vi "Periodic Tasks.vi"(8 "error in":errorcluster) -> ()   [LabVIEW 2015]
doc: "This VI runs in parallel to other tasks. It can contain as many user-defined periodic loops as you need. These can carry out PID or other sorts of timed response."
uses:
  <vilib>/Rock Robotics/WPI/DriverStation/WPI_DriverStationRobotMode2.ctl
  <vilib>/Rock Robotics/WPI/Solenoid/WPI_SolenoidValue.ctl
  <vilib>/Rock Robotics/WPI/Utilities/WPI_GetSetVariantRefNum.vi
  Robot Global Data.vi
  <vilib>/Rock Robotics/WPI/Solenoid/WPI_SolenoidSetEnum.vi
  <vilib>/Rock Robotics/Network Tables/NT Write Boolean.vi
  <vilib>/Rock Robotics/Network Tables/NT Write Number.vi
  <vilib>/Rock Robotics/Network Tables/NT Read Boolean.vi
  NavX/navX Library v2/navX Library v2.lvlib
panel:
  out "12 (Shooter angle)":dbl
  out "Shooter 2":dbl
  out "Shooter 1":dbl
  out "Energy (J)":dbl
  out "Power (W)":dbl
  out "15":dbl
  out "0":dbl
  out "14":dbl
  out "1":dbl
  out "current (A)":dbl
  out "Loop Time":u32
  in  "Roll":dbl=3.0
  in  "Pitch":dbl=3.0
  out "Value":bool
  out "Enum":T1(ring)
  out "isFlat":bool
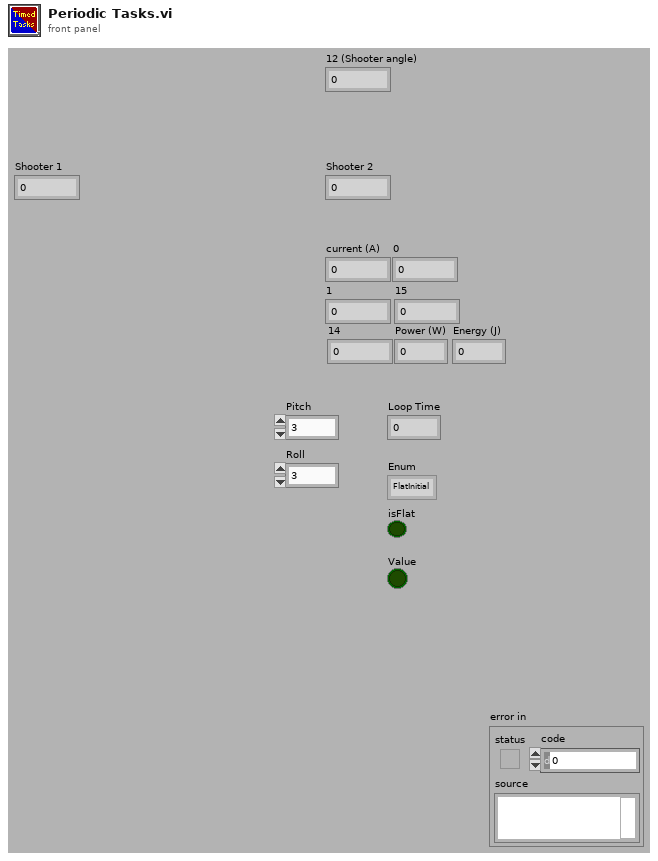
[diagram p1: front panel]
types:
  T1 = enum16{"FlatInitial", "AngleUp", "AngleDown", "FlatFinal"}
  T2 = typedef "WPI_RobotDriveDevRef.ctl" = cluster{"DevStatus":errorcluster, "Motors[]":T3[], "Square Inputs":bool, "Max Output":dbl}
  T3 = typedef "WPI_MotorControlDeviceRef.ctl" = cluster{"DeviceStatus":errorcluster, "Type":T4, "PWM":cluster{"PWM Channel":T5, "DeadBand":T6}, "CAN":cluster{"Device Number":u8, "Control Mode":T7, "Semaphore":T8, "Max Vout":dbl, "TalonSRX Control Mode":T9}, "Invert":bool}
  T4 = typedef "WPI_MotorControlType.ctl" = enum16{"PWM", "CAN", "CANTalonSRX"}
  T5 = typedef "FPGA_DIOPWMChannel.ctl" = enum8{"PWM 0", "PWM 1", "PWM 2", "PWM 3", "PWM 4", "PWM 5", "PWM 6", "PWM 7", "PWM 8", "PWM 9", "PWM MXP 0", "PWM MXP 1", "PWM MXP 2", "PWM MXP 3", "PWM MXP 4", "PWM MXP 5", "PWM MXP 6", "PWM MXP 7", "PWM MXP 8", "PWM MXP 9", "Invalid"}
  T6 = typedef "WPI_PWMDeadband.ctl" = cluster{"Name":string, "maxPositivePwm":i32, "minPositivePwm":i32, "centerPwm":i32, "maxNegativePwm":i32, "minNegativePwm":i32, "angularRange":u16}
  T7 = typedef "WPI_CANJaguar_ControlMode.ctl" = enum8{"Percent VBus", "Current", "Speed", "Position", "Voltage"}
  T8 = typedef "Semaphore RefNum" = refnum<k1>
  T9 = typedef "WPI_CANTalonSRX_APIControlMode.ctl" = enum8{"Percent VBus", "Speed", "Position", "Slave", "Unchanged / Invalid", "Voltage Compensation", "Current", "Motion Profile"}
  T10 = typedef "WPI_DigitalInputDevRef.ctl" = cluster{"DevStatus":errorcluster, "DIO Channel":T11}
  T11 = typedef "FPGA_DIOChannel.ctl" = enum8{"DIO 0", "DIO 1", "DIO 2", "DIO 3", "DIO 4", "DIO 5", "DIO 6", "DIO 7", "DIO 8", "DIO 9", "DIO MXP 0", "DIO MXP 1", "DIO MXP 2", "DIO MXP 3", "DIO MXP 4", "DIO MXP 5", "DIO MXP 6", "DIO MXP 7", "DIO MXP 8", "DIO MXP 9", "DIO MXP 10", "DIO MXP 11", "DIO MXP 12", "DIO MXP 13", "DIO MXP 14", "DIO MXP 15", "Invalid"}
  T12 = typedef "WPI_SolenoidDevRef.ctl" = cluster{"DevStatus":errorcluster, "Pneumatics Control Module":u8, "Forward Solenoid Channel":T13, "Reverse Solenoid Channel":T13}
  T13 = typedef "WPI_SolenoidChannel.ctl" = enum8{"Solenoid 0", "Solenoid 1", "Solenoid 2", "Solenoid 3", "Solenoid 4", "Solenoid 5", "Solenoid 6", "Solenoid 7", "Invalid"}
  T14 = typedef "WPI_EncoderDevRef.ctl" = cluster{"DevStatus":errorcluster, "EncoderIndex":T15, "CounterIndex":T16, "DistancePerCount":dbl, "Decoding Type":T17}
  T15 = typedef "FPGA_EncoderIdx.ctl" = enum8{"Enc 0", "Enc 1", "Enc 2", "Enc 3", "Enc 4", "Enc 5", "Enc 6", "Enc 7", "Invalid"}
  T16 = typedef "FPGA_CounterCtrSystemIndex.ctl" = enum8{"Ctr 0", "Ctr 1", "Ctr 2", "Ctr 3", "Ctr 4", "Ctr 5", "Ctr 6", "Ctr 7", "Invalid"}
  T17 = typedef "WPI_EncoderType.ctl" = enum16{"1x", "2x", "4x"}
  T18 = typedef "navX Library v2.lvlib/Z900_navX_DeviceTypeDef.ctl" = cluster{"Interface":cluster{"Protocol":T19, "Update Rate (4Hz-60Hz)":u8, "navX Open TypeDef":variant}, "Notify Packet":refnum<notifier>, "Loop VI Refnum":refnum<vi>, "Ready to Close Occurrence Refnum":refnum<k4>}
  T19 = typedef "navX Library v2.lvlib/Z900_navX_ProtocolTypeDef.ctl" = enum16{"SERIAL", "I2C", "SPI"}
  T20 = typedef "WPI_SolenoidValue.ctl" = enum16{"Off", "On", "Forward", "Reverse"}
  T21 = typedef "WPI_DriverStationRobotMode2.ctl" = enum16{"Autonomous Disabled", "Autonomous Enabled", "Teleop Disabled", "Teleop Enabled", "Disconnected", "Finish", "Test Disabled", "Test Enabled", "Emergency Stopped"}
  T22 = typedef "WPI_GyroDevRef.ctl" = cluster{"DevStatus":errorcluster, "Analog Channel":T23, "Offset":dbl, "Gain (VoltsPerDegree/Second)":dbl, "Gyro Type":enum16{"Analog", "XRS450"}, "Handle":i32, "SPI Bus":T24, "Device Found":bool, "Sample Rate":dbl, "Calibrate On Open":bool}
  T23 = typedef "FPGA_AIChannel.ctl" = enum8{"AI 0", "AI 1", "AI 2", "AI 3", "AI MXP 0", "AI MXP 1", "AI MXP 2", "AI MXP 3", "Invalid"}
  T24 = typedef "spi_bus.ctl" = enum16{"SPI On-Board, CS0", "SPI On-Board, CS1", "SPI On-Board, CS2", "SPI On-Board, CS3", "SPI MXP", "Invalid"}
  T25 = cluster{"Velocity X":dbl, "Velocity Y":dbl, "Velocity Z":dbl, "Displacement X":dbl, "Displacement Y":dbl, "Displacement Z":dbl}
  T26 = cluster{"Yaw":dbl, "Roll":dbl, "Pitch":dbl, "Heading":dbl, "Fused Heading":dbl}
  T27 = enum16{"Empty", "Suck", "Hold", "LowGoal", "HighGoal", "BumperShot", "Shoot", "Dwell"}
  T28 = enum16{"ResetBack", "EmergencyManualControl", "ResetForward", "Hold", "Reset", "ManualControl"}
  T29 = cluster{"LinearAcceleration X":dbl, "LinearAcceleration Y":dbl, "LinearAcceleration Z":dbl}
  T30 = enum16{"ResetBack", "ResetForward", "Reset", "Hold", "HighGoal", "LowGoal", "BumperShot", "EmergencyManualControl"}
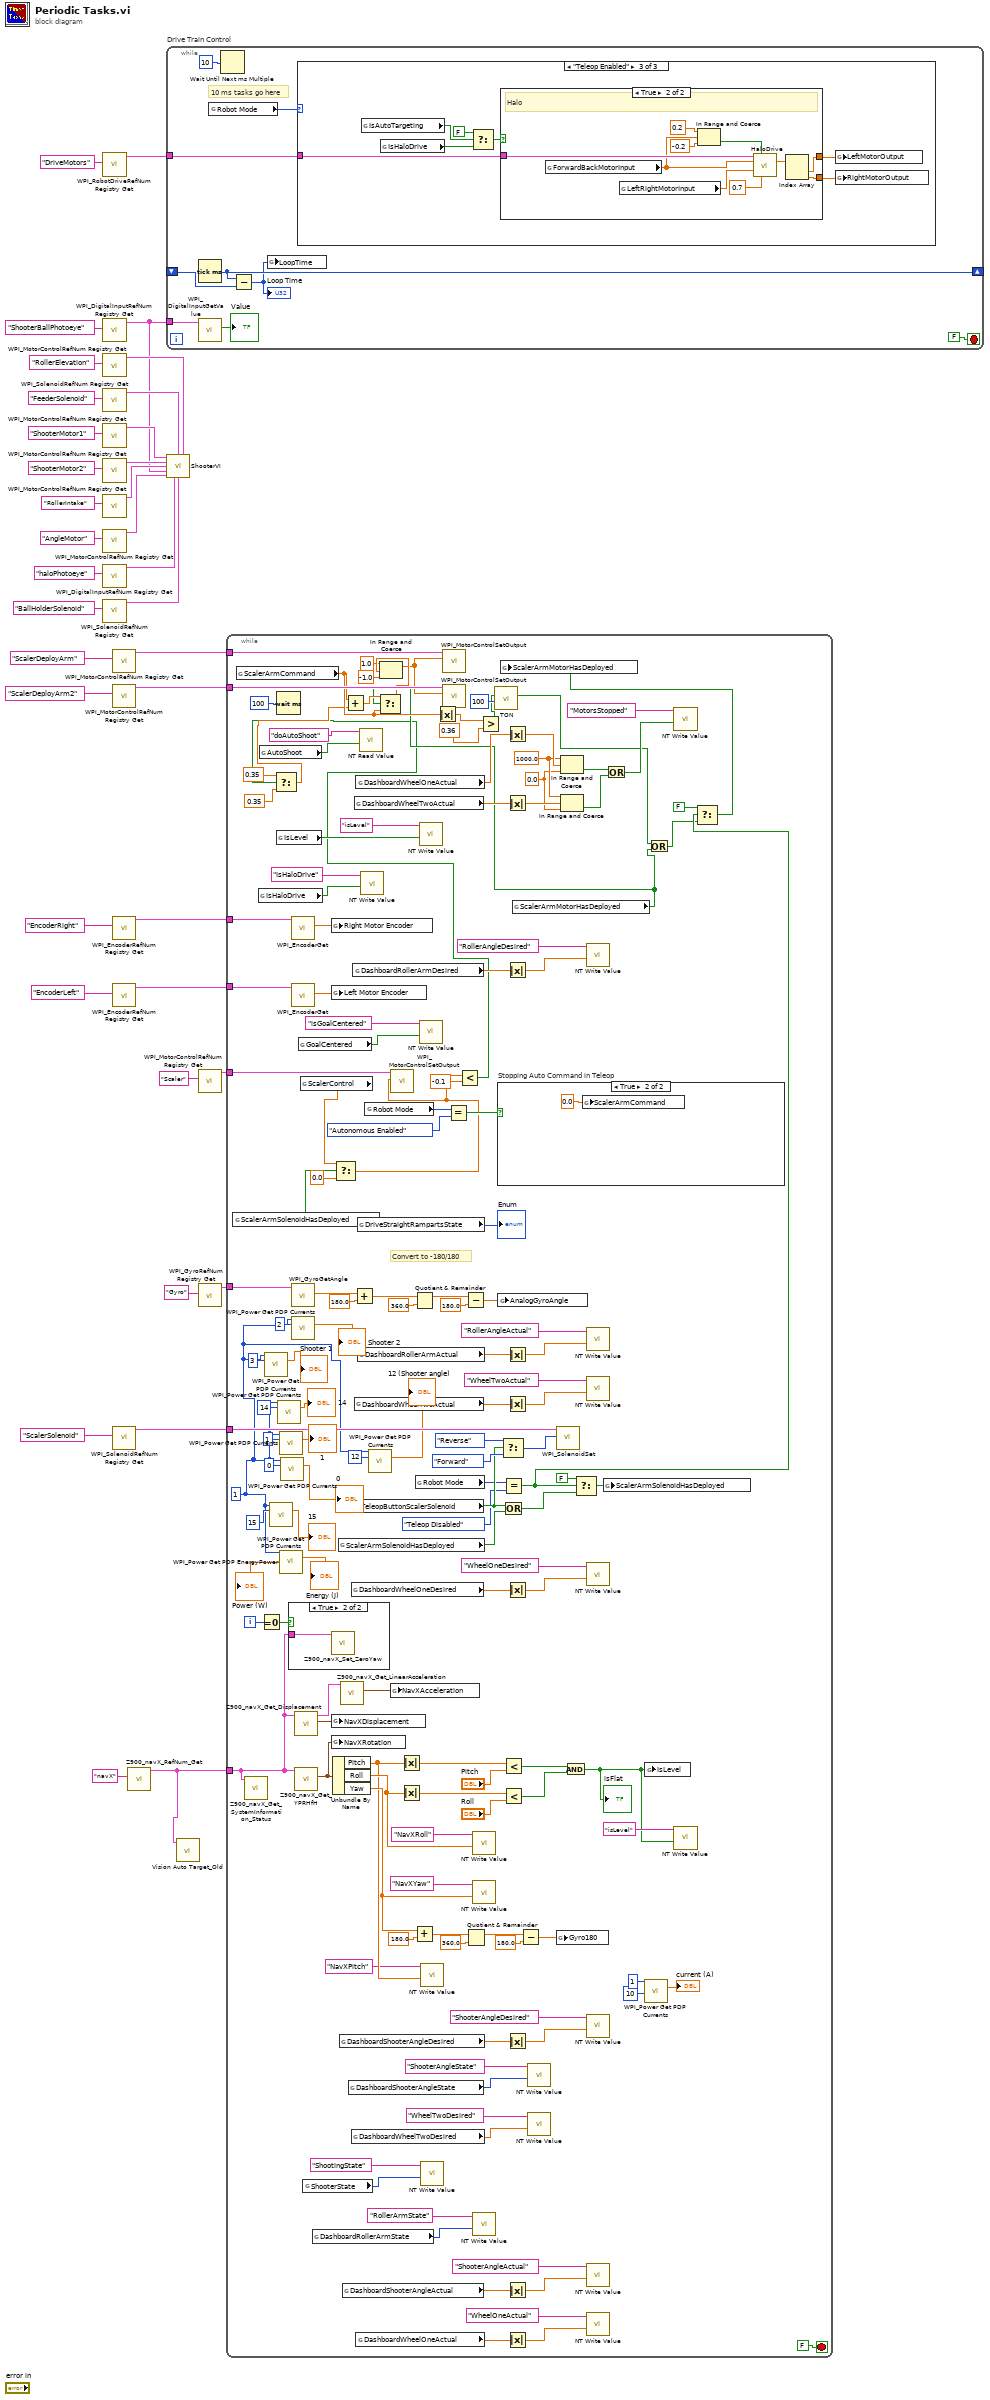
[diagram p0: block diagram]
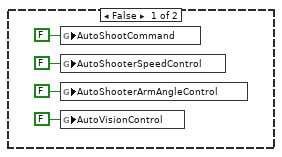
[diagram p2: hidden frame]
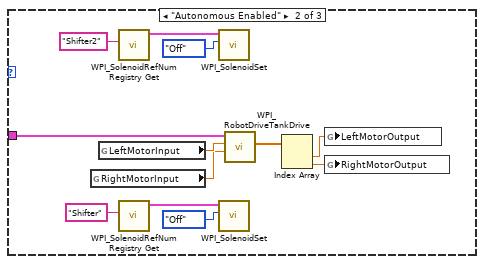
[diagram p5: hidden frame]
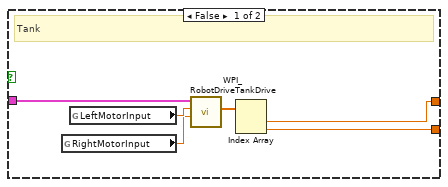
[diagram p6: hidden frame]
diagram:
  n1 = call <vilib>:"WPI_RobotDriveRefNum Registry Get.vi"("refnum name"="DriveMotors") -> ("RobotDriveDevRef"=w35:T2)  [unwired: 9 in, 1 out]
  n2 = call <vilib>:"WPI_DigitalInputRefNum Registry Get.vi"("refnum name"="ShooterBallPhotoeye") -> ("DigitalInputDevRef"=w1:T10)  [unwired: 9 in, 1 out]
  n3 = call <vilib>:"WPI_MotorControlRefNum Registry Get.vi"("refnum name"="RollerElevation") -> ("MotorControlDevRef"=w23:T3)  [unwired: 9 in, 1 out]
  n4 = call <vilib>:"WPI_SolenoidRefNum Registry Get.vi"("refnum name"="FeederSolenoid") -> ("SolenoidDevRef"=w19:T12)  [unwired: 9 in, 1 out]
  n5 = call <vilib>:"WPI_MotorControlRefNum Registry Get.vi"("refnum name"="ShooterMotor1") -> ("MotorControlDevRef"=w22:T3)  [unwired: 9 in, 1 out]
  n6 = call <vilib>:"WPI_MotorControlRefNum Registry Get.vi"("refnum name"="ShooterMotor2") -> ("MotorControlDevRef"=w21:T3)  [unwired: 9 in, 1 out]
  n7 = call <vilib>:"WPI_MotorControlRefNum Registry Get.vi"("refnum name"="RollerIntake") -> ("MotorControlDevRef"=w20:T3)  [unwired: 9 in, 1 out]
  n8 = call <vilib>:"WPI_MotorControlRefNum Registry Get.vi"("refnum name"="AngleMotor") -> ("MotorControlDevRef"=w17:T3)  [unwired: 9 in, 1 out]
  n9 = call <vilib>:"WPI_DigitalInputRefNum Registry Get.vi"("refnum name"="haloPhotoeye") -> ("DigitalInputDevRef"=w3:T10)  [unwired: 9 in, 1 out]
  n10 = call <vilib>:"WPI_SolenoidRefNum Registry Get.vi"("refnum name"="BallHolderSolenoid") -> ("SolenoidDevRef"=w10:T12)  [unwired: 9 in, 1 out]
  n11 = call <vilib>:"WPI_MotorControlRefNum Registry Get.vi"("refnum name"="ScalerDeployArm") -> ("MotorControlDevRef"=w16:T3)  [unwired: 9 in, 1 out]
  n12 = call <vilib>:"WPI_MotorControlRefNum Registry Get.vi"("refnum name"="ScalerDeployArm2") -> ("MotorControlDevRef"=w5:T3)  [unwired: 9 in, 1 out]
  n13 = call <vilib>:"WPI_EncoderRefNum Registry Get.vi"("refnum name"="EncoderRight") -> ("EncoderDevRef"=w31:T14)  [unwired: 9 in, 1 out]
  n14 = call <vilib>:"WPI_EncoderRefNum Registry Get.vi"("refnum name"="EncoderLeft") -> ("EncoderDevRef"=w32:T14)  [unwired: 9 in, 1 out]
  n15 = call <vilib>:"WPI_SolenoidRefNum Registry Get.vi"("refnum name"="ScalerSolenoid") -> ("SolenoidDevRef"=w7:T12)  [unwired: 9 in, 1 out]
  n16 = call "Z900_navX_RefNum_Get.vi"("refnum name"="navX") -> ("navX Device"=w2:T18)  [unwired: 9 in, 1 out]
  n17 = while "Drive Train Control" {
    tunnel: w35 -> [w44]
    tunnel: w1 -> [w42]
    shift-right: [w39] -> _
    shift-left: _ -> [w40]
    stop <- FALSE stop-if-true
    # "10 ms tasks go here"
    n18 = Tick Count (ms)() -> (millisecond timer value=w39:u32)
    n19 = call <vilib>:"WPI_DigitalInputGetValue.vi"("DigitalInputDevRef"=w42) -> ("Value"=→"Value":bool)  [unwired: 8 in, 2 out]
    n20 = global read "Robot Global Data.vi" "Robot Mode"() -> (w43:T21)
    n21 = Wait Until Next ms Multiple(millisecond multiple=u32 10 ("milliseconds to wait")) -> ()  [unwired: 1 out]
    n22 = Subtract(x=w39, y=w40) -> (x-y=w38:u32)
    "Loop Time" <- w38
    n23 = global write "Robot Global Data.vi" "LoopTime"(w38) -> ()
    n24 = case shown="\"Teleop Enabled\"" w43 {
      tunnel: w44 -> [_ w57 w64]
      frame "Autonomous Disabled", "Teleop Disabled", Default {
      }
      frame "Autonomous Enabled" {
        n25 = global read "Robot Global Data.vi" "RightMotorInput"() -> (w49:dbl)
        n26 = global read "Robot Global Data.vi" "LeftMotorInput"() -> (w50:dbl)
        n27 = call <vilib>:"WPI_SolenoidRefNum Registry Get.vi"("refnum name"="Shifter2") -> ("SolenoidDevRef"=w52:T12)  [unwired: 9 in, 1 out]
        n28 = call <vilib>:"WPI_SolenoidRefNum Registry Get.vi"("refnum name"="Shifter") -> ("SolenoidDevRef"=w51:T12)  [unwired: 9 in, 1 out]
        n29 = call-poly <vilib>:"WPI_SolenoidSet.vi"("Value"=WPI_SolenoidValue."Off", "SolenoidDevRef"=w52) -> ()  [unwired: 8 in, 2 out]
        n30 = call-poly <vilib>:"WPI_SolenoidSet.vi"("Value"=WPI_SolenoidValue."Off", "SolenoidDevRef"=w51) -> ()  [unwired: 8 in, 2 out]
        n31 = call <vilib>:"WPI_RobotDriveTankDrive.vi"("Right axis value"=w49, "Left axis value"=w50, "RobotDriveDevRef"=w57) -> ("Motor Values"=w48:dbl[])  [unwired: 6 in, 2 out]
        n32 = Index Array(array=w48) -> (element #1=w47:dbl, element #2=w46:dbl)  [unwired: 2 in]
        n33 = global write "Robot Global Data.vi" "LeftMotorOutput"(w47) -> ()
        n34 = global write "Robot Global Data.vi" "RightMotorOutput"(w46) -> ()
      }
      frame "Teleop Enabled" {
        n35 = global read "Robot Global Data.vi" "IsAutoTargeting"() -> (w61:bool)
        n36 = global read "Robot Global Data.vi" "IsHaloDrive"() -> (w59:bool)
        n37 = Select(t=FALSE, s=w61, f=w59) -> (s? t:f=w58:bool)
        n38 = case shown="True" w58 {
          tunnel: w64 -> [w68 w80]
          tunnel: [w67 w72] -> w63
          tunnel: [w66 w71] -> w62
          frame False {
            # "Tank"
            n39 = global read "Robot Global Data.vi" "RightMotorInput"() -> (w69:dbl)
            n40 = global read "Robot Global Data.vi" "LeftMotorInput"() -> (w70:dbl)
            n41 = call <vilib>:"WPI_RobotDriveTankDrive.vi"("Right axis value"=w69, "Left axis value"=w70, "RobotDriveDevRef"=w68) -> ("Motor Values"=w65:dbl[])  [unwired: 6 in, 2 out]
            n42 = Index Array(array=w65) -> (element #1=w67:dbl, element #2=w66:dbl)  [unwired: 2 in]
          }
          frame True {
            # "Halo"
            n43 = global read "Robot Global Data.vi" "ForwardBackMotorInput"() -> (w74:dbl)
            n44 = global read "Robot Global Data.vi" "LeftRightMotorInput"() -> (w75:dbl)
            n45 = In Range and Coerce(upper limit=0.2, x=w74, lower limit=-0.2) -> (In Range?=w76:bool)  [unwired: 1 out]
            n46 = call "HaloDrive.vi"("RobotDriveDevRef 2"=w80, "QwikTurnButton"=w76, "Left axis value"=w74, "Right axis value"=w75, "Sensitivity"=0.7) -> ("Motor Values"=w73:dbl[])  [unwired: 6 in, 4 out]
            n47 = Index Array(array=w73) -> (element #1=w72:dbl, element #2=w71:dbl)  [unwired: 2 in]
          }
        }
        n48 = global write "Robot Global Data.vi" "LeftMotorOutput"(w63) -> ()
        n49 = global write "Robot Global Data.vi" "RightMotorOutput"(w62) -> ()
      }
    }
  }
  n50 = call "ShooterVI.vi"("Shooter Motor 1"=w22, "ShooterSolenoid"=w19, "Roller Angle Motor"=w23, "Shooter Motor 2"=w21, "Roller Intake Motor"=w20, "Ball Detector Photoeye"=w1, "ShooterAngleMotor"=w17, "Halo Photoeye"=w3, "BallHolderSolenoid"=w10) -> ()  [unwired: 7 in]
  n51 = call "Vision Auto Target_Old.vi"("navX Device"=w2) -> ()  [unwired: 11 in]
  n52 = call <vilib>:"WPI_MotorControlRefNum Registry Get.vi"("refnum name"="Scaler") -> ("MotorControlDevRef"=w14:T3)  [unwired: 9 in, 1 out]
  n53 = call <vilib>:"WPI_GyroRefNum Registry Get.vi"("refnum name"="Gyro") -> ("GyroDevRef"=w13:T22)  [unwired: 9 in, 1 out]
  n54 = while {
    tunnel: w32 -> [w228]
    tunnel: w31 -> [w229]
    tunnel: w2 -> [w150]
    tunnel: w16 -> [w173]
    tunnel: w14 -> [w172]
    tunnel: w13 -> [w158]
    tunnel: w7 -> [w146]
    tunnel: w5 -> [w145]
    i -> [w225]
    stop <- FALSE stop-if-true
    w83 = u8 1 ("Power Distribution Panel (0)")
    w139 = 0.0 ("lower limit")
    w140 = 1000.0
    # "Convert to -180/180"
    n55 = global read "Robot Global Data.vi" "ScalerArmSolenoidHasDeployed"() -> (w125:bool)
    n56 = global read "Robot Global Data.vi" "ScalerArmCommand"() -> (w112:dbl)
    n57 = call "Z900_navX_Get_SystemInformation_Status.vi"("navX Device"=w150) -> ()  [unwired: 7 in, 4 out]
    n58 = global read "Robot Global Data.vi" "IsHaloDrive"() -> (w226:bool)
    n59 = global read "Robot Global Data.vi" "AutoShoot"() -> (w185:bool)
    n60 = Equal To 0?(x=w225) -> (x = 0?=w224:bool)
    n61 = call <vilib>:"WPI_Power Get PDP Currents.vi"("Power Distribution Panel (0)"=w83, "PDP Channel"=3) -> ("current (A)"=→"Shooter 1":dbl)  [unwired: 11 in, 2 out]
    n62 = call <vilib>:"WPI_Power Get PDP Currents.vi"("Power Distribution Panel (0)"=w83, "PDP Channel"=15) -> ("current (A)"=→"15":dbl)  [unwired: 11 in, 2 out]
    n63 = global read "Robot Global Data.vi" "IsLevel"() -> (w183:bool)
    n64 = Wait (ms)(milliseconds to wait=u32 100) -> ()  [unwired: 1 out]
    n65 = call <vilib>:"WPI_Power Get PDP Currents.vi"("Power Distribution Panel (0)"=w83, "PDP Channel"=14) -> ("current (A)"=→"14":dbl)  [unwired: 11 in, 2 out]
    n66 = call <vilib>:"WPI_Power Get PDP Currents.vi"("Power Distribution Panel (0)"=w83, "PDP Channel"=1) -> ("current (A)"=→"1":dbl)  [unwired: 11 in, 2 out]
    n67 = call <vilib>:"WPI_Power Get PDP EnergyPower.vi"("Power Distribution Panel (0)"=w83) -> ("Energy (J)"=→"Energy (J)":dbl, "Power (W)"=→"Power (W)":dbl)  [unwired: 12 in, 1 out]
    n68 = call <vilib>:"WPI_Power Get PDP Currents.vi"("Power Distribution Panel (0)"=w83, "PDP Channel"=0) -> ("current (A)"=→"0":dbl)  [unwired: 11 in, 2 out]
    n69 = case shown="True" w224 {
      tunnel: w150 -> [_ w237]
      frame False {
      }
      frame True {
        n70 = call "Z900_navX_Set_ZeroYaw.vi"("navX Device"=w237) -> ()  [unwired: 9 in, 2 out]
      }
    }
    n71 = call <vilib>:"WPI_EncoderGet.vi"("EncoderDevRef"=w229) -> ("Distance"=w149:dbl)  [unwired: 5 in, 5 out]
    n72 = call <vilib>:"WPI_EncoderGet.vi"("EncoderDevRef"=w228) -> ("Distance"=w148:dbl)  [unwired: 5 in, 5 out]
    n73 = call <vilib>:"WPI_GyroGetAngle.vi"("GyroDevRef"=w158) -> ("Angle"=w152:dbl)  [unwired: 6 in, 4 out]
    n74 = call <vilib>:"WPI_Power Get PDP Currents.vi"("Power Distribution Panel (0)"=w83, "PDP Channel"=2) -> ("current (A)"=→"Shooter 2":dbl)  [unwired: 11 in, 2 out]
    n75 = call "Z900_navX_Get_Displacement.vi"("navX Device"=w150) -> ("Displacement"=w218:T25, "navX Device"=w216:T18)  [unwired: 7 in, 2 out]
    n76 = call "Z900_navX_Get_YPRHfH.vi"("navX Device"=w150) -> ("YRPHfH"=w223:T26)  [unwired: 7 in, 3 out]
    n77 = global read "Robot Global Data.vi" "GoalCentered"() -> (w187:bool)
    n78 = global read "Robot Global Data.vi" "ScalerControl"() -> (w123:dbl)
    n79 = global read "Robot Global Data.vi" "ShooterState"() -> (w204:T27)
    n80 = global read "Robot Global Data.vi" "DashboardRollerArmState"() -> (w203:T28)
    n81 = global write "Robot Global Data.vi" "Right Motor Encoder"(w149) -> ()
    n82 = global write "Robot Global Data.vi" "Left Motor Encoder"(w148) -> ()
    n83 = global write "Robot Global Data.vi" "NavXDisplacement"(w218) -> ()
    n84 = global write "Robot Global Data.vi" "NavXRotation"(w223) -> ()
    n85 = Unbundle By Name(w223) -> ("Pitch"=w175:dbl, "Roll"=w177:dbl, "Yaw"=w179:dbl)
    n86 = Select(t=w123, s=w125, f=0.0) -> (s? t:f=w106:dbl)
    n87 = global read "Robot Global Data.vi" "ScalerArmSolenoidHasDeployed"() -> (w131:bool)
    n88 = global read "Robot Global Data.vi" "DashboardShooterAngleDesired"() -> (w196:dbl)
    n89 = call "Z900_navX_Get_LinearAcceleration.vi"("navX Device"=w216) -> ("Linear Acceleration"=w217:T29)  [unwired: 7 in, 3 out]
    n90 = global read "Robot Global Data.vi" "DashboardShooterAngleActual"() -> (w195:dbl)
    n91 = global read "Robot Global Data.vi" "DashboardShooterAngleState"() -> (w202:T30)
    n92 = global read "Robot Global Data.vi" "DashboardWheelOneDesired"() -> (w201:dbl)
    n93 = global read "Robot Global Data.vi" "DashboardWheelTwoDesired"() -> (w199:dbl)
    n94 = global read "Robot Global Data.vi" "DashboardRollerArmDesired"() -> (w198:dbl)
    n95 = Add(x=w152, y=180.0) -> (x+y=w156:dbl)
    n96 = global read "Robot Global Data.vi" "TeleopButtonScalerSolenoid"() -> (w132:bool)
    n97 = global read "Robot Global Data.vi" "DashboardWheelTwoActual"() -> (w143:dbl)
    n98 = global read "Robot Global Data.vi" "DashboardWheelTwoActual"() -> (w194:dbl)
    n99 = global read "Robot Global Data.vi" "DashboardWheelOneActual"() -> (w144:dbl)
    n100 = global read "Robot Global Data.vi" "DashboardWheelOneActual"() -> (w200:dbl)
    n101 = global read "Robot Global Data.vi" "DriveStraightRampartsState"() -> (→"Enum":T1)
    n102 = global read "Robot Global Data.vi" "DashboardRollerArmActual"() -> (w197:dbl)
    n103 = call-poly <vilib>:"NT Read Value.vi"("Default Value"=w185, "Name"="doAutoShoot") -> ()  [unwired: 8 in, 2 out]
    n104 = call-poly <vilib>:"NT Write Value.vi"("Boolean"=w226, "Name"="IsHaloDrive") -> ()  [unwired: 9 in, 1 out]
    n105 = global read "Robot Global Data.vi" "Robot Mode"() -> (w169:T21)
    n106 = call <vilib>:"WPI_Power Get PDP Currents.vi"("Power Distribution Panel (0)"=w83, "PDP Channel"=12) -> ("current (A)"=→"12 (Shooter angle)":dbl)  [unwired: 11 in, 2 out]
    n107 = call <vilib>:"WPI_MotorControlSetOutput.vi"("Output"=w106, "MotorControlDevRef"=w172) -> ()  [unwired: 7 in, 3 out]
    n108 = global write "Robot Global Data.vi" "NavXAcceleration"(w217) -> ()
    n109 = Absolute Value(x=w175) -> (abs(x)=w222:dbl)
    n110 = Absolute Value(x=w177) -> (abs(x)=w220:dbl)
    n111 = Add(x=w179, y=180.0) -> (x+y=w192:dbl)
    n112 = Quotient & Remainder(x=w156, y=360.0) -> (x-y*floor(x/y)=w154:dbl)  [unwired: 1 out]
    n113 = global read "Robot Global Data.vi" "Robot Mode"() -> (w130:T21)
    n114 = call-poly <vilib>:"NT Write Value.vi"("Boolean"=w183, "Name"="isLevel") -> ()  [unwired: 9 in, 1 out]
    n115 = call-poly <vilib>:"NT Write Value.vi"("Boolean"=w187, "Name"="isGoalCentered") -> ()  [unwired: 9 in, 1 out]
    n116 = call-poly <vilib>:"NT Write Value.vi"("Numeric"=w175, "Name"="NavXPitch") -> ()  [unwired: 9 in, 1 out]
    n117 = call-poly <vilib>:"NT Write Value.vi"("Numeric"=w204, "Name"="ShootingState") -> ()  [unwired: 9 in, 1 out]
    n118 = Absolute Value(x=w112) -> (abs(x)=w114:dbl)
    n119 = Equal?(x=w169, y=WPI_DriverStationRobotMode2."Autonomous Enabled") -> (x = y?=w167:bool)
    n120 = Less?(x=w106, y=-0.1) -> (x < y?=w99:bool)
    n121 = Select(t=0.35, s=w99, f=0.35 ("y")) -> (s? t:f=w103:dbl)
    n122 = Add(x=w112, y=w103) -> (x+y=w113:dbl)
    n123 = Subtract(x=w154, y=180.0) -> (x-y=w151:dbl)
    n124 = Quotient & Remainder(x=w192, y=360.0) -> (x-y*floor(x/y)=w190:dbl)  [unwired: 1 out]
    n125 = call-poly <vilib>:"NT Write Value.vi"("Numeric"=w177, "Name"="NavXRoll") -> ()  [unwired: 9 in, 1 out]
    n126 = call-poly <vilib>:"NT Write Value.vi"("Numeric"=w179, "Name"="NavXYaw") -> ()  [unwired: 9 in, 1 out]
    n127 = call-poly <vilib>:"NT Write Value.vi"("Numeric"=w203, "Name"="RollerArmState") -> ()  [unwired: 9 in, 1 out]
    n128 = Greater?(x=w114, y=0.36 ("upper limit")) -> (0:w116:bool)
    n129 = call "TON.vi"("Delay (ms)"=u32 100, "Input"=w116) -> ("Output"=w121:bool)  [unwired: 9 in]
    n130 = case "Stopping Auto Command in Teleop" shown="True" w167 {
      frame False {
        n131 = global write "Robot Global Data.vi" "AutoShootCommand"(FALSE ("AutoShooterSpeedControl")) -> ()
        n132 = global write "Robot Global Data.vi" "AutoShooterSpeedControl"(FALSE ("AutoShooterSpeedControl")) -> ()
        n133 = global write "Robot Global Data.vi" "AutoShooterArmAngleControl"(FALSE ("AutoShooterSpeedControl")) -> ()
        n134 = global write "Robot Global Data.vi" "AutoVisionControl"(FALSE ("AutoVisionControl")) -> ()
      }
      frame True {
        n135 = global write "Robot Global Data.vi" "ScalerArmCommand"(0.0 ("ScalerArmCommand")) -> ()
      }
    }
    n136 = global write "Robot Global Data.vi" "AnalogGyroAngle"(w151) -> ()
    n137 = Select(t=WPI_SolenoidValue."Reverse" ("Value"), s=w132, f=WPI_SolenoidValue."Forward") -> (s? t:f=w133:T20)
    n138 = Equal?(x=w130, y=WPI_DriverStationRobotMode2."Teleop Disabled") -> (x = y?=w120:bool)
    n139 = Or(x=w132, y=w131) -> (x .or. y?=w128:bool)
    n140 = Less?(x=w222, y="Pitch") -> (x < y?=w221:bool)
    n141 = Less?(x=w220, y="Roll") -> (x < y?=w219:bool)
    n142 = Absolute Value(x=w144) -> (abs(x)=w142:dbl)
    n143 = Absolute Value(x=w143) -> (abs(x)=w141:dbl)
    n144 = Absolute Value(x=w198) -> (abs(x)=w159:dbl)
    n145 = Absolute Value(x=w197) -> (abs(x)=w163:dbl)
    n146 = Absolute Value(x=w194) -> (abs(x)=w160:dbl)
    n147 = Absolute Value(x=w201) -> (abs(x)=w161:dbl)
    n148 = Absolute Value(x=w196) -> (abs(x)=w162:dbl)
    n149 = Absolute Value(x=w195) -> (abs(x)=w165:dbl)
    n150 = Absolute Value(x=w200) -> (abs(x)=w164:dbl)
    n151 = global read "Robot Global Data.vi" "ScalerArmMotorHasDeployed"() -> (w111:bool)
    n152 = Select(t=w113, s=w111, f=w112) -> (s? t:f=w110:dbl)
    n153 = In Range and Coerce(upper limit=1.0, x=w110, lower limit=-1.0) -> (coerced(x)=w107:dbl)  [unwired: 1 out]
    n154 = call <vilib>:"WPI_MotorControlSetOutput.vi"("Output"=w107, "MotorControlDevRef"=w173) -> ()  [unwired: 7 in, 3 out]
    n155 = call <vilib>:"WPI_MotorControlSetOutput.vi"("Output"=w107, "MotorControlDevRef"=w145) -> ()  [unwired: 7 in, 3 out]
    n156 = Subtract(x=w190, y=180.0) -> (x-y=w188:dbl)
    n157 = call-poly <vilib>:"NT Write Value.vi"("Numeric"=w202, "Name"="ShooterAngleState") -> ()  [unwired: 9 in, 1 out]
    n158 = call-poly <vilib>:"NT Write Value.vi"("Numeric"=w199, "Name"="WheelTwoDesired") -> ()  [unwired: 9 in, 1 out]
    n159 = call-poly <vilib>:"WPI_SolenoidSet.vi"("Value"=w133, "SolenoidDevRef"=w146) -> ()  [unwired: 8 in, 2 out]
    n160 = global write "Robot Global Data.vi" "Gyro180"(w188) -> ()
    n161 = In Range and Coerce(upper limit=w140, x=w142, lower limit=w139) -> (In Range?=w137:bool)  [unwired: 1 out]
    n162 = In Range and Coerce(upper limit=w140, x=w141, lower limit=w139) -> (In Range?=w138:bool)  [unwired: 1 out]
    n163 = And(x=w221, y=w219) -> (x .and. y?=w170:bool)
    "isFlat" <- w170
    n164 = Select(t=FALSE, s=w120, f=w128) -> (s? t:f=w126:bool)
    n165 = call-poly <vilib>:"NT Write Value.vi"("Numeric"=w159, "Name"="RollerAngleDesired") -> ()  [unwired: 9 in, 1 out]
    n166 = call-poly <vilib>:"NT Write Value.vi"("Numeric"=w163, "Name"="RollerAngleActual") -> ()  [unwired: 9 in, 1 out]
    n167 = call-poly <vilib>:"NT Write Value.vi"("Numeric"=w160, "Name"="WheelTwoActual") -> ()  [unwired: 9 in, 1 out]
    n168 = call-poly <vilib>:"NT Write Value.vi"("Numeric"=w161, "Name"="WheelOneDesired") -> ()  [unwired: 9 in, 1 out]
    n169 = call-poly <vilib>:"NT Write Value.vi"("Numeric"=w162, "Name"="ShooterAngleDesired") -> ()  [unwired: 9 in, 1 out]
    n170 = call-poly <vilib>:"NT Write Value.vi"("Numeric"=w165, "Name"="ShooterAngleActual") -> ()  [unwired: 9 in, 1 out]
    n171 = call-poly <vilib>:"NT Write Value.vi"("Numeric"=w164, "Name"="WheelOneActual") -> ()  [unwired: 9 in, 1 out]
    n172 = global write "Robot Global Data.vi" "ScalerArmSolenoidHasDeployed"(w126) -> ()
    n173 = Or(x=w137, y=w138) -> (x .or. y?=w135:bool)
    n174 = call <vilib>:"WPI_Power Get PDP Currents.vi"("Power Distribution Panel (0)"=u8 1, "PDP Channel"=10) -> ("current (A)"=→"current (A)":dbl)  [unwired: 11 in, 2 out]
    n175 = global write "Robot Global Data.vi" "IsLevel"(w170) -> ()
    n176 = Or(x=w121, y=w111) -> (x .or. y?=w119:bool)
    n177 = call-poly <vilib>:"NT Write Value.vi"("Boolean"=w135, "Name"="MotorsStopped") -> ()  [unwired: 9 in, 1 out]
    n178 = call-poly <vilib>:"NT Write Value.vi"("Boolean"=w170, "Name"="isLevel") -> ()  [unwired: 9 in, 1 out]
    n179 = Select(t=FALSE, s=w120, f=w119) -> (s? t:f=w117:bool)
    n180 = global write "Robot Global Data.vi" "ScalerArmMotorHasDeployed"(w117) -> ()
  }
